vi "Get Optimal Plane.vi"(0 "Image Src (RGB)":T2, 2 "ROI Descriptor":T1, 11 "Error in (no error)":errorcluster) -> (3 "Maximum Standard Deviation":sgl, 4 "Color Plane to be Extracted":i32(ring)=7 items=["Red", "Green", "Blue", "Hue", "Saturation", "Luminance", "Value", "Intensity"], 15 "Error out":errorcluster)   [LabVIEW 2025]
uses:
  <vilib>/vision/Image Controls.llb/IMAQ Image.ctl
  <vilib>/Utility/error.llb/Error Cluster From Error Code.vi
  <vilib>/ErrorRing/Error Ring.xnode
  <vilib>/vision/NI_Vision_Development_Module.lvlib
panel:
  out "Standard Variation Vector":sgl[](array[numeric])
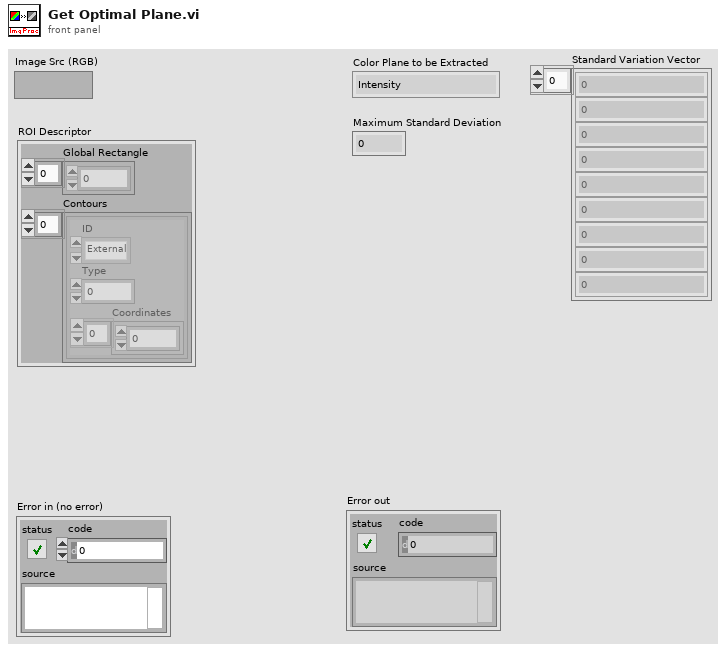
[diagram p1: front panel]
types:
  T1 = cluster{"Global Rectangle":i32[], "Contours":cluster{"ID":enum32{"External", "Internal"}, "Type":u32, "Coordinates":i32[]}[]}
  T2 = typedef "IMAQ Image.ctl" = refnum<image>
  T3 = typedef "Image Type" = u32
  T4 = cluster{"histogram":u32[], "Minimal Value":sgl, "Maximal Value":sgl, "Starting Value":sgl, "Interval Width":sgl, "Mean Value":sgl, "Standard  Variation":sgl, "Area (pixels)":i32}
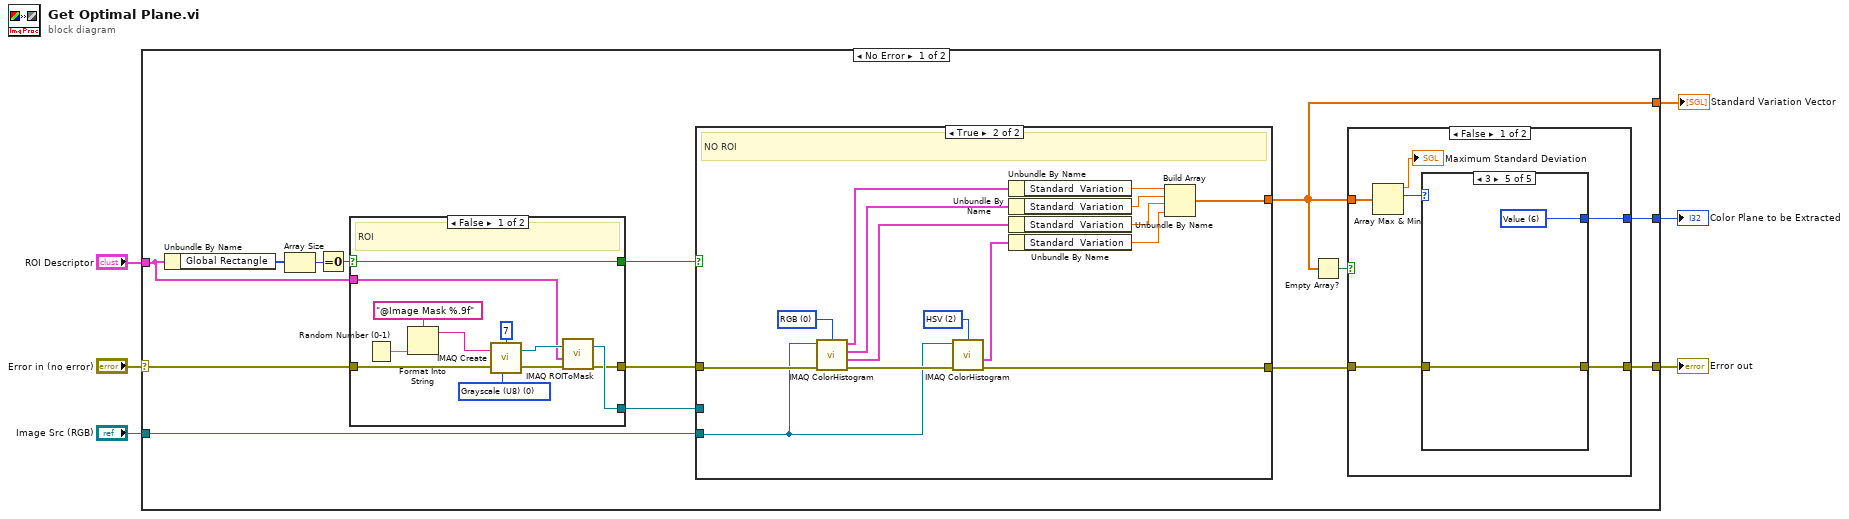
[diagram p0: block diagram]
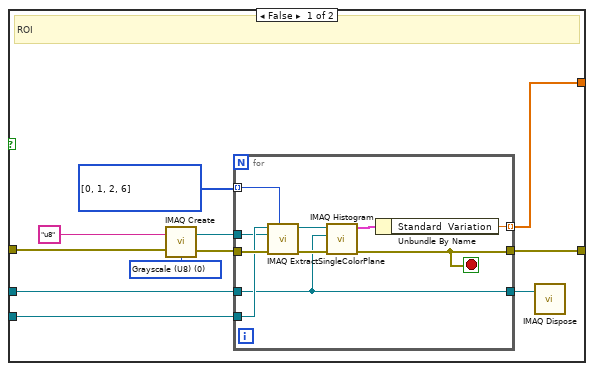
[diagram p2: hidden frame]
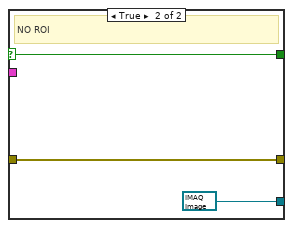
[diagram p3: hidden frame]
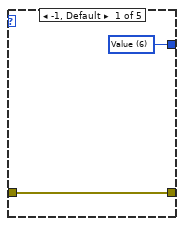
[diagram p4: hidden frame]
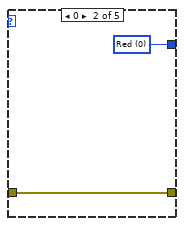
[diagram p5: hidden frame]
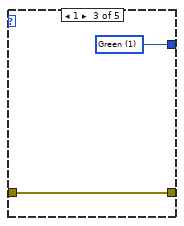
[diagram p6: hidden frame]
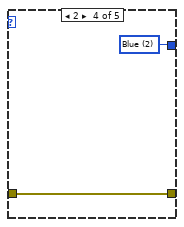
[diagram p7: hidden frame]
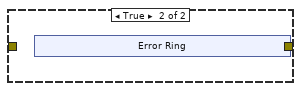
[diagram p8: hidden frame]
diagram:
  n1 = case shown="No Error" "Error in (no error)" {
    selector: "Error in (no error)" -> [w12 _]
    tunnel: "Image Src (RGB)" -> [w20 _]
    tunnel: [w17 _] -> w4
    tunnel: [w19 _] -> w3
    tunnel: [w16 _] -> w2
    tunnel: "ROI Descriptor" -> [w13 _]
    frame No Error {
      n2 = Unbundle By Name(w13) -> ("Global Rectangle"=w10:i32[])
      n3 = Array Size(array=w10) -> (size(s)=w14:i32)
      n4 = Equal To 0?(x=w14) -> (x = 0?=w15:bool)
      n5 = case shown="False" w15 {
        selector: w15 -> [w57 w69]
        tunnel: [w65 T2 refnum ("Image Out")] -> w9
        tunnel: w13 -> [w61 _]
        tunnel: w12 -> [w60 w70]
        tunnel: [w58 w70] -> w11
        tunnel: [w57 w69] -> w7
        frame False {
          w66 = T3 0 items=["Grayscale (U8)", "Grayscale (I16)", "Grayscale (SGL)", "Complex (CSG)", "RGB (U32)", "HSL (U32)", "RGB (U64)", "Grayscale (U16)"] ("Image Type")
          # "ROI"
          n6 = Random Number (0-1)() -> (number: 0 to 1=w62:dbl)
          n7 = Format Into String(format string="@Image Mask %.9f" ("Image Name"), w62) -> (resulting string=w64:string)  [unwired: 2 in, 1 out]
          n8 = call "IMAQ Create"("Border Size"=7, "Image Name"=w64, "Image Type"=w66, "error in (no error)"=w60) -> ("New Image"=w68:T2, "error out"=w59:errorcluster)  [unwired: 1 out]
          n9 = call "IMAQ ROIToMask"("error in (no error)"=w59, "ROI Descriptor"=w61, "Image"=w68) -> ("error out"=w58:errorcluster, "Image Out"=w65:T2)  [unwired: 2 in, 2 out]
        }
        frame True {
          # "NO ROI"
        }
      }
      n10 = case shown="True" w7 {
        tunnel: w20 -> [w31 w43]
        tunnel: [w30 w42] -> w16
        tunnel: w11 -> [w29 w44]
        tunnel: w9 -> [w28 _]
        tunnel: [w27 w45] -> w8
        frame False {
          w24 = T3 0 items=["Grayscale (U8)", "Grayscale (I16)", "Grayscale (SGL)", "Complex (CSG)", "RGB (U32)", "HSL (U32)", "RGB (U64)", "Grayscale (U16)"] ("Image Type")
          w26 = i32[] [0, 1, 2, 6] items=["Red", "Green", "Blue", "Hue", "Saturation", "Luminance", "Value", "Intensity"] ("Color Plane")
          # "ROI"
          n11 = call "IMAQ Create"("Image Name"="u8", "Image Type"=w24, "error in (no error)"=w29) -> ("New Image"=w23:T2, "error out"=w25:errorcluster)  [unwired: 2 in]
          n12 = for {
            tunnel: w26 -> [w39] mode=indexing
            tunnel: [w37] -> w30 mode=indexing
            tunnel: w25 -> [w36]
            tunnel: [w34] -> w27
            tunnel: w31 -> [w35]
            tunnel: w28 -> [w32]
            tunnel: w23 -> [w33]
            tunnel: [w32] -> w22
            stop <- w34 stop-if-true
            n13 = call "IMAQ ExtractSingleColorPlane"("Color Plane"=w39, "error in (no error)"=w36, "Image Dst"=w33, "Image Src"=w35) -> ("error out"=w40:errorcluster, "Image Dst Out"=w41:T2)  [unwired: 6 in]
            n14 = call "IMAQ Histogram"("error in (no error)"=w40, "Image Mask"=w32, "Image"=w41) -> ("error out"=w34:errorcluster, "Histogram Report"=w38:T4)  [unwired: 7 in]
            n15 = Unbundle By Name(w38) -> ("Standard  Variation"=w37:sgl)
          }
          n16 = call "IMAQ Dispose"("Image"=w22) -> ()  [unwired: 5 in, 1 out]
        }
        frame True {
          w49 = u16 2 items=["RGB", "HSL", "HSV", "HSI", "CIE L*a*b*", "CIE XYZ"] ("Color Mode")
          w56 = u16 0 items=["RGB", "HSL", "HSV", "HSI", "CIE L*a*b*", "CIE XYZ"] ("Color Mode")
          # "NO ROI"
          n17 = call "IMAQ ColorHistogram"("Color Mode"=w56, "Image Src"=w43, "error in (no error)"=w44) -> ("Red or Hue or X or L* Histogram Report"=w55:T4, "Green or Sat or Y or a* Histogram Report"=w54:T4, "Blue or Luma or Val or Inten or Z or b* Histogram Report"=w53:T4, "error out"=w46:errorcluster)  [unwired: 3 in]
          n18 = call "IMAQ ColorHistogram"("Color Mode"=w49, "Image Src"=w43, "error in (no error)"=w46) -> ("Blue or Luma or Val or Inten or Z or b* Histogram Report"=w48:T4, "error out"=w45:errorcluster)  [unwired: 3 in, 2 out]
          n19 = Unbundle By Name(w55) -> ("Standard  Variation"=w52:sgl)
          n20 = Unbundle By Name(w54) -> ("Standard  Variation"=w51:sgl)
          n21 = Unbundle By Name(w53) -> ("Standard  Variation"=w50:sgl)
          n22 = Unbundle By Name(w48) -> ("Standard  Variation"=w47:sgl)
          n23 = Build Array(w52, w51, w50, w47) -> (w42:sgl[])
        }
      }
      n24 = Empty Array?(array=w16) -> (empty?=w18:bool)
      n25 = case shown="False" w18 {
        tunnel: [w76 _] -> w19
        tunnel: w16 -> [w75 _]
        tunnel: w8 -> [w74 _]
        tunnel: [w73 w88] -> w17
        frame False {
          n26 = Array Max & Min(array=w75) -> (max value=→"Maximum Standard Deviation":sgl, max index (indices)=w77:i32)  [unwired: 2 out]
          n27 = case shown="3" w77 {
            tunnel: [w79 w81 w83 w85 w87] -> w76
            tunnel: w74 -> [w78 w80 w82 w84 w86]
            tunnel: [w78 w80 w82 w84 w86] -> w73
            frame -1, Default {
              w79 = 6 items=["Red", "Green", "Blue", "Hue", "Saturation", "Luminance", "Value", "Intensity"] ("Color Plane")
            }
            frame 0 {
              w81 = 0 items=["Red", "Green", "Blue", "Hue", "Saturation", "Luminance", "Value", "Intensity"] ("Color Plane")
            }
            frame 1 {
              w83 = 1 items=["Red", "Green", "Blue", "Hue", "Saturation", "Luminance", "Value", "Intensity"] ("Color Plane")
            }
            frame 2 {
              w85 = 2 items=["Red", "Green", "Blue", "Hue", "Saturation", "Luminance", "Value", "Intensity"] ("Color Plane")
            }
            frame 3 {
              w87 = 6 items=["Red", "Green", "Blue", "Hue", "Saturation", "Luminance", "Value", "Intensity"] ("Color Plane")
            }
          }
        }
        frame True {
          n28 = xnode "Error Ring"() -> ("error out"=w88:errorcluster)
        }
      }
    }
    frame Error {
    }
  }
  "Error out" <- w4
  "Color Plane to be Extracted" <- w3
  "Standard Variation Vector" <- w2
